vi "Calibrate load cells.vi"() -> (3 "Slope and Intercept":dbl[][](array[numeric]))   [LabVIEW 2015]
uses:
  <vilib>/Utility/file.llb/Write Delimited Spreadsheet (DBL).vi
  <vilib>/Analysis/NI_AALPro.lvlib
  <vilib>/gmath/NI_Gmath.lvlib
panel:
  out "Left Hindlimb":dbl[](array[numeric])
  out "Right Hindlimb":dbl[](array[numeric])
  out "Forelimb":dbl[](array[numeric])
  in  "?":bool
  in  "Tab Control":T1(tab)
  in  "200g":bool
  out "200g":dbl
  in  "100g":bool
  out "100g":dbl
  in  "50g":bool
  out "50g":dbl
  in  "OK Button":bool
  out "10g":dbl
  out "5g":dbl
  out "2g":dbl
  out "0g":dbl
  in  "20g":bool
  in  "15g":bool
  in  "10g":bool
  in  "2g":bool
  in  "0g":bool
  in  "5g":bool
  out "15g":dbl
  out "20g":dbl
  out "20g HR":dbl
  out "15g HR":dbl
  in  "5g HR":bool
  in  "0g HR":bool
  in  "2g HR":bool
  in  "10g HR":bool
  in  "15g HR":bool
  in  "20g HR":bool
  out "0g HR":dbl
  out "2g HR":dbl
  out "5g HR":dbl
  out "10g HR":dbl
  in  "OK Button 2":bool
  out "50g HR":dbl
  in  "50g HR":bool
  out "100g HR":dbl
  in  "100g HR":bool
  out "200g HR":dbl
  in  "200g HR":bool
  out "20g LH":dbl
  out "15g HL":dbl
  in  "5g HL":bool
  in  "0g HL":bool
  in  "2g HL":bool
  in  "10g HL":bool
  in  "15g HL":bool
  in  "20g HL":bool
  out "0g HL":dbl
  out "2g HL":dbl
  out "5g HL":dbl
  out "10g HL":dbl
  in  "OK Button 3":bool
  out "50g HL":dbl
  in  "50g HL":bool
  out "100g HL":dbl
  in  "100g HL":bool
  out "200g HL":dbl
  in  "200g HL":bool
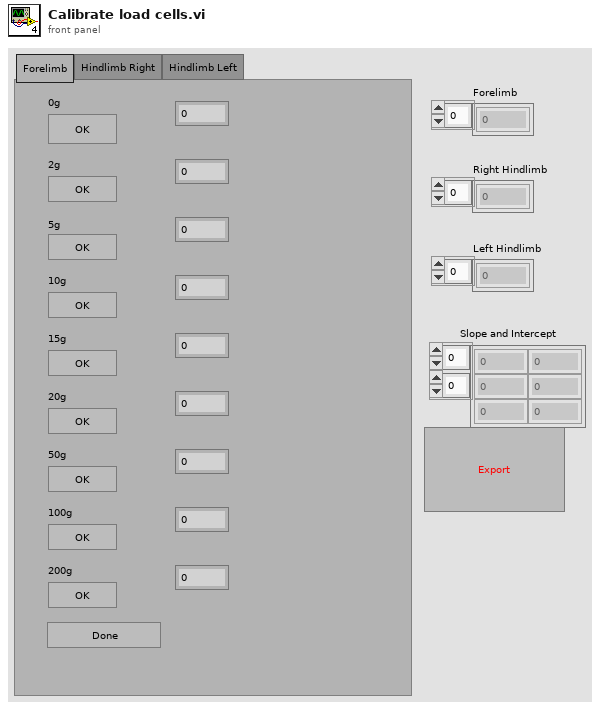
[diagram p1: front panel]
types:
  T1 = enum32{"Forelimb", "Hindlimb Right", "Hindlimb Left"}
  T2 = enum16{"arithmetic", "geometric", "harmonic", "trimmed", "median"}
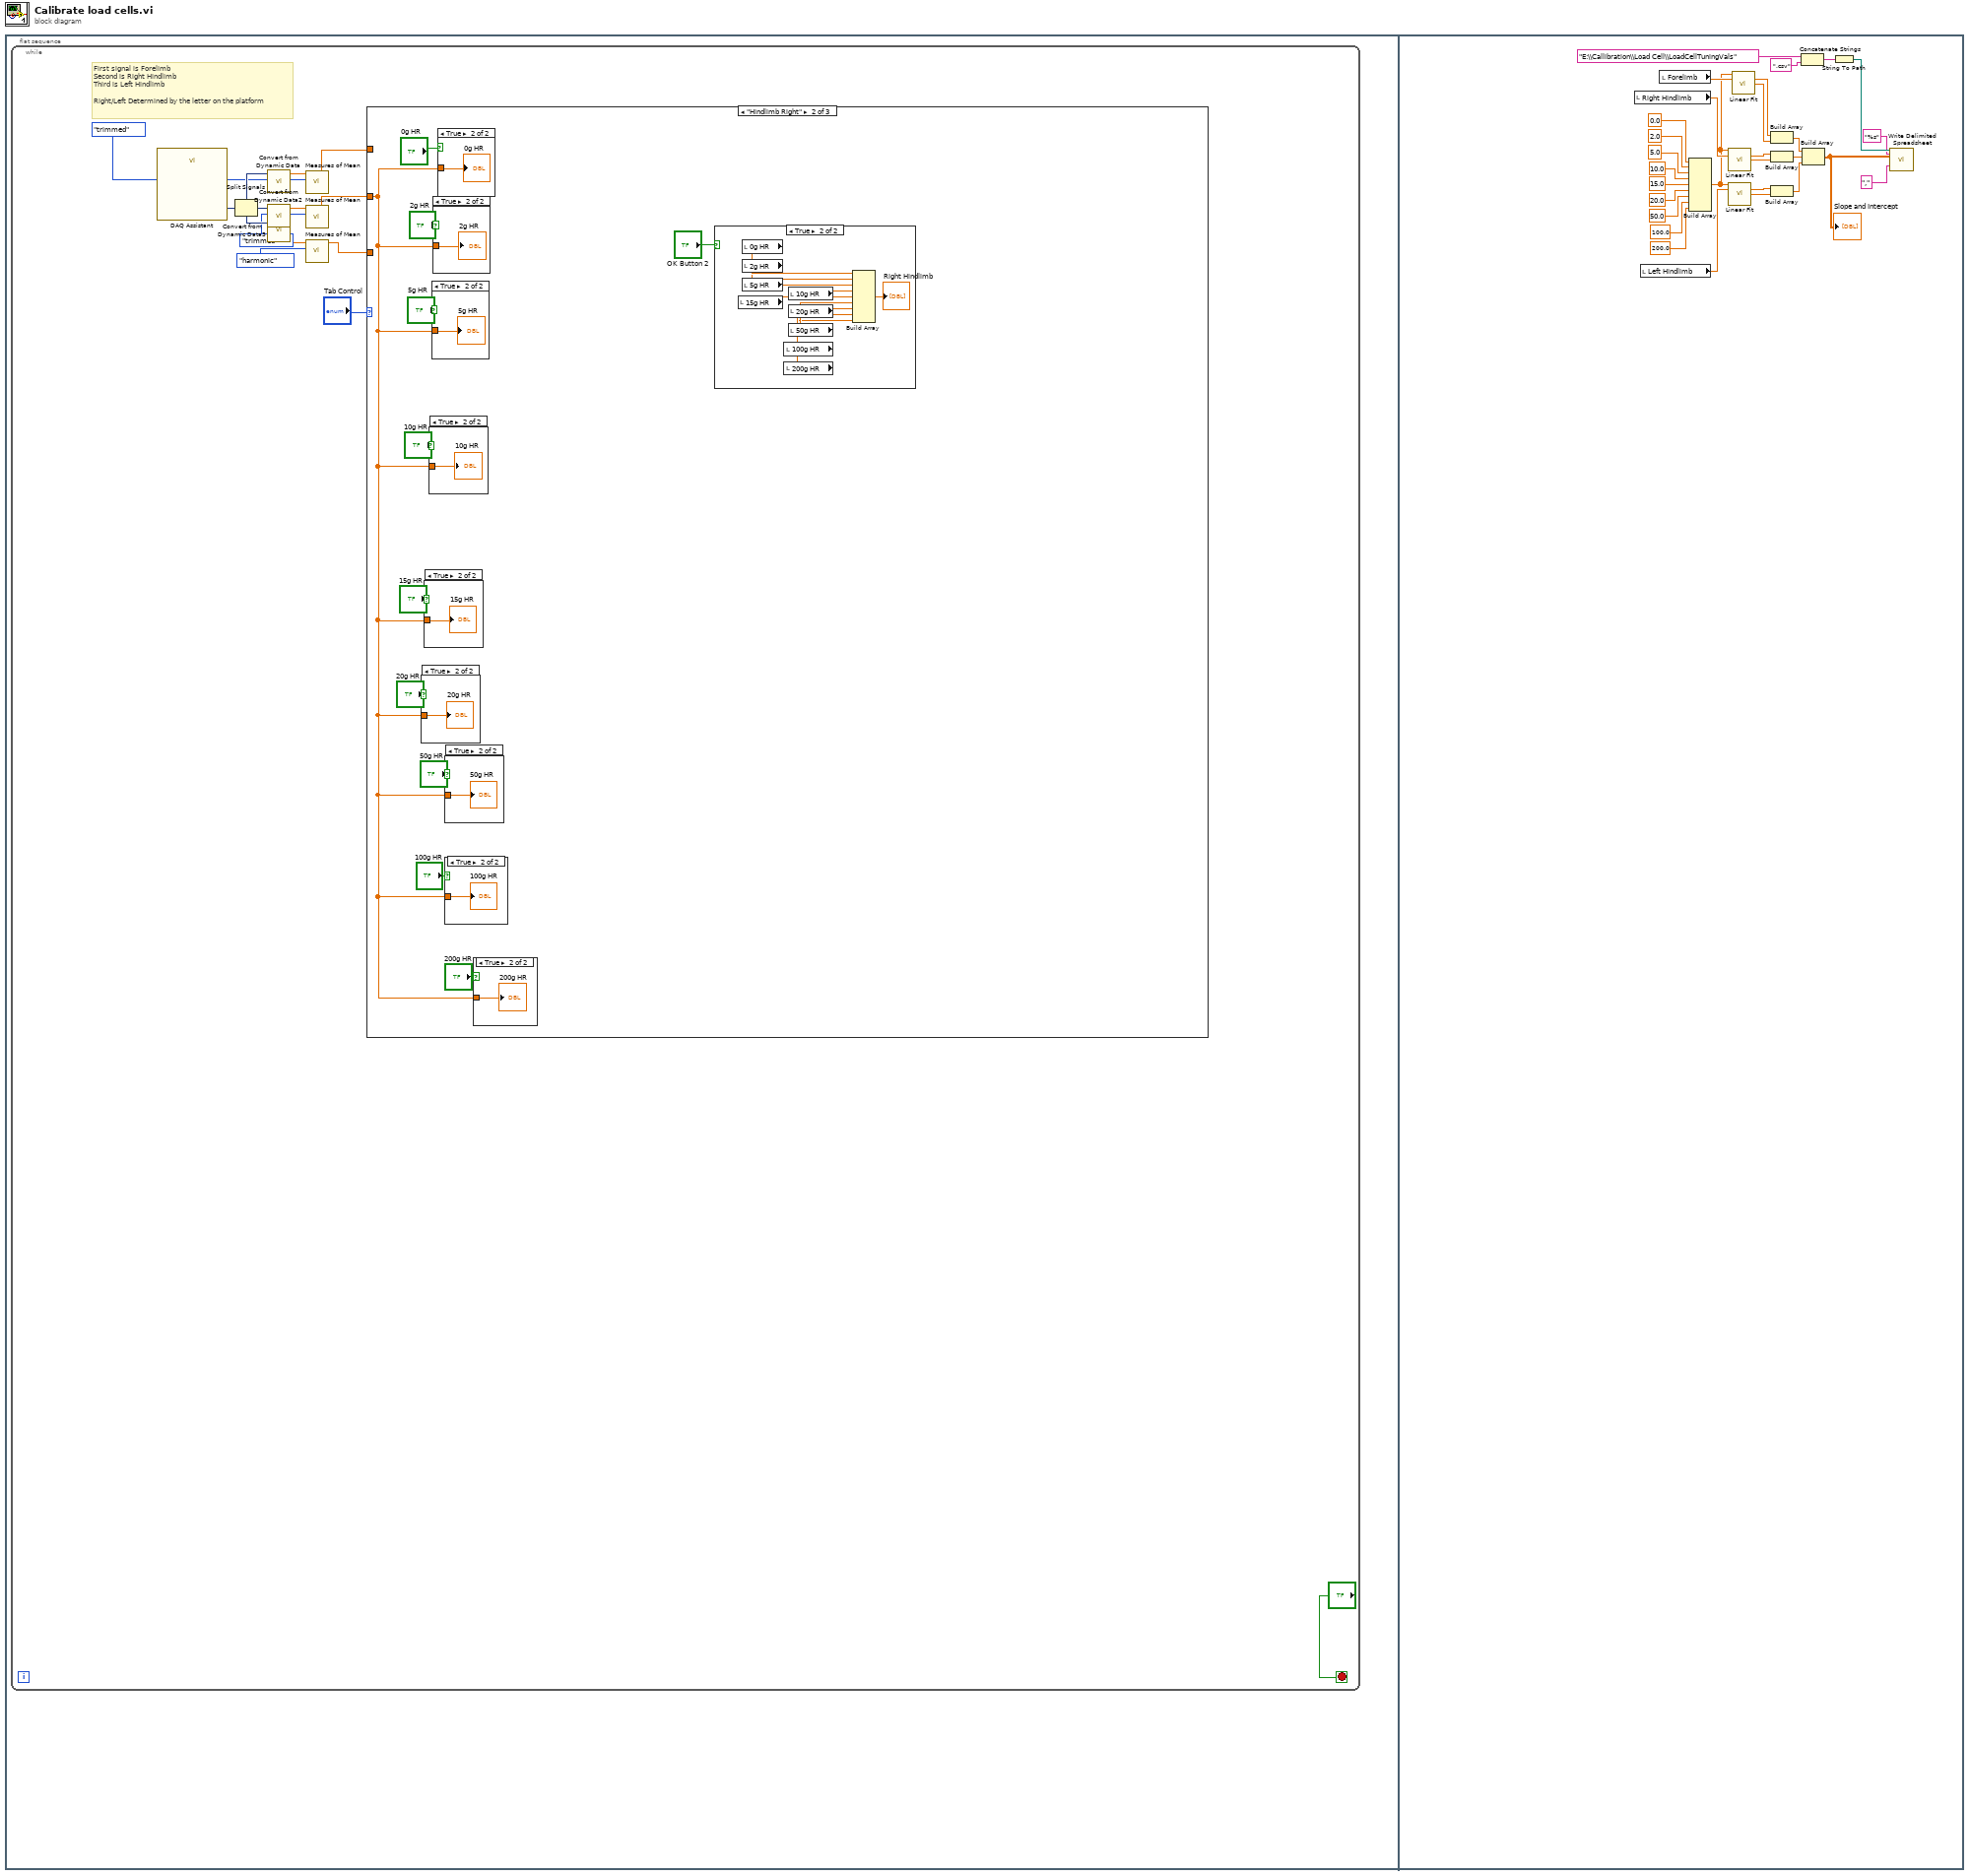
[diagram p0: block diagram]
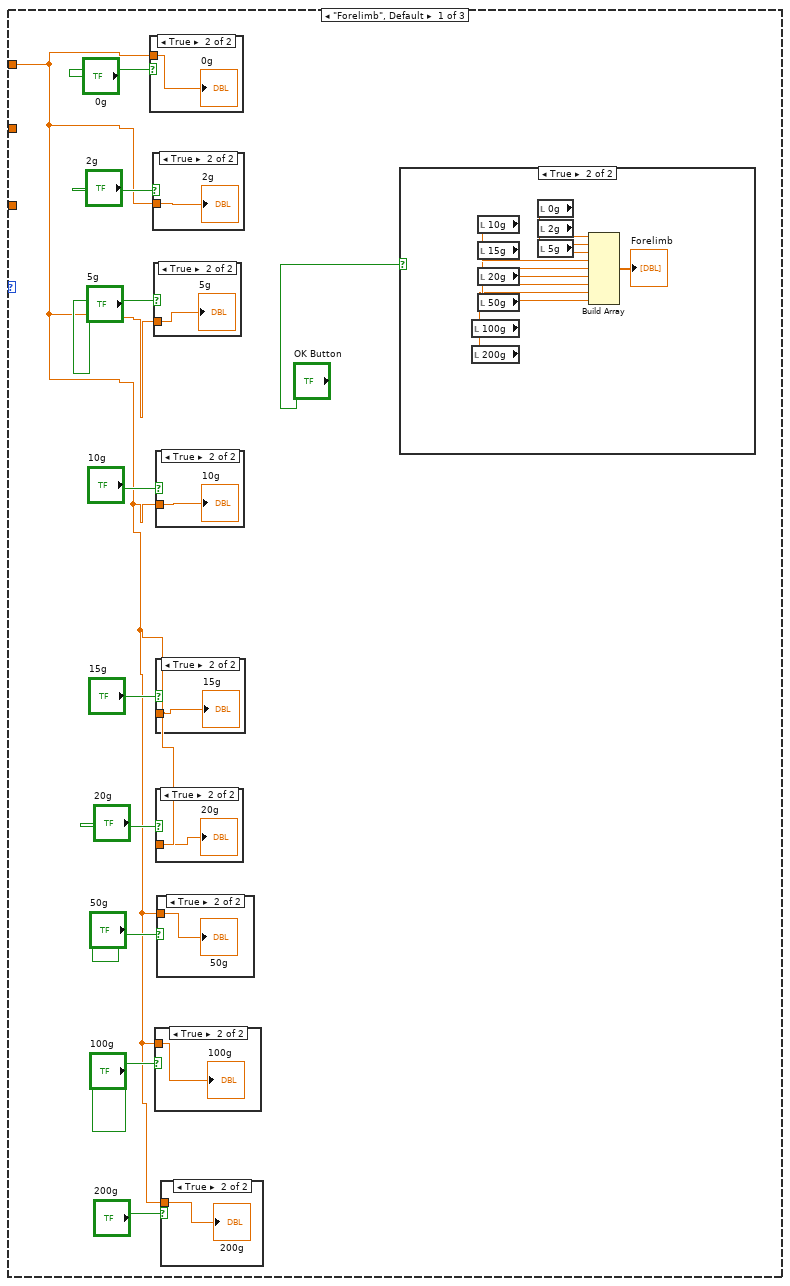
[diagram p2: hidden frame]
diagram:
  n1 = flat-sequence {
    frame #0 {
      n2 = while {
        stop <- "?" stop-if-true
        # "First signal is Forelimb\nSecond is Right Hindlimb\nThird is Left Hindlimb\n\nRight/Left Determined by the letter on the platform"
        n3 = call "DAQ Assistant"() -> ("data"=w7:dynamicdata)  [unwired: 17 in, 2 out]
        n4 = Split Signals(w7) -> (w15:dynamicdata, w13:dynamicdata, w11:dynamicdata)  [unwired: 3 in]
        n5 = call "Convert from Dynamic Data"("Dynamic Data Type"=w15) -> ("Array"=w14:dbl[])  [unwired: 3 in]
        n6 = call "Convert from Dynamic Data2"("Dynamic Data Type"=w13) -> ("Array"=w12:dbl[])  [unwired: 3 in]
        n7 = call "Convert from Dynamic Data3"("Dynamic Data Type"=w11) -> ("Array"=w6:dbl[])  [unwired: 3 in]
        n8 = call <vilib>:"Measures of Mean.vi"("type"=T2."trimmed", "x array"=w14) -> ("mean value"=w9:dbl)  [unwired: 8 in, 1 out]
        n9 = call <vilib>:"Measures of Mean.vi"("type"=T2."trimmed", "x array"=w12) -> ("mean value"=w2:dbl)  [unwired: 8 in, 1 out]
        n10 = call <vilib>:"Measures of Mean.vi"("type"=T2."harmonic", "x array"=w6) -> ("mean value"=w1:dbl)  [unwired: 8 in, 1 out]
        n11 = case shown="\"Hindlimb Right\"" "Tab Control" {
          tunnel: w9 -> [w16 _ _]
          tunnel: w1 -> [_ _ w76]
          tunnel: w2 -> [_ w46 _]
          frame "Forelimb", Default {
            n12 = case shown="True" "0g" {
              tunnel: w16 -> [_ w45]
              frame False {
              }
              frame True {
                "0g" <- w45
              }
            }
            n13 = case shown="True" "2g" {
              tunnel: w16 -> [_ w44]
              frame False {
              }
              frame True {
                "2g" <- w44
              }
            }
            n14 = case shown="True" "5g" {
              tunnel: w16 -> [_ w43]
              frame False {
              }
              frame True {
                "5g" <- w43
              }
            }
            n15 = case shown="True" "100g" {
              tunnel: w16 -> [_ w28]
              frame False {
              }
              frame True {
                "100g" <- w28
              }
            }
            n16 = case shown="True" "10g" {
              tunnel: w16 -> [_ w42]
              frame False {
              }
              frame True {
                "10g" <- w42
              }
            }
            n17 = case shown="True" "15g" {
              tunnel: w16 -> [_ w41]
              frame False {
              }
              frame True {
                "15g" <- w41
              }
            }
            n18 = case shown="True" "20g" {
              tunnel: w16 -> [_ w40]
              frame False {
              }
              frame True {
                "20g" <- w40
              }
            }
            n19 = case shown="True" "50g" {
              tunnel: w16 -> [_ w29]
              frame False {
              }
              frame True {
                "50g" <- w29
              }
            }
            n20 = case shown="True" "200g" {
              tunnel: w16 -> [_ w27]
              frame False {
              }
              frame True {
                "200g" <- w27
              }
            }
            n21 = case shown="True" "OK Button" {
              frame False {
              }
              frame True {
                n22 = local read "100g"() -> (w31:dbl)
                n23 = local read "200g"() -> (w30:dbl)
                n24 = local read "10g"() -> (w36:dbl)
                n25 = local read "15g"() -> (w35:dbl)
                n26 = local read "20g"() -> (w34:dbl)
                n27 = local read "50g"() -> (w32:dbl)
                n28 = local read "0g"() -> (w39:dbl)
                n29 = local read "2g"() -> (w38:dbl)
                n30 = local read "5g"() -> (w37:dbl)
                n31 = Build Array(w39, w38, w37, w36, w35, w34, w32, w31, w30) -> (→"Forelimb":dbl[])
              }
            }
          }
          frame "Hindlimb Right" {
            n32 = case shown="True" "20g HR" {
              tunnel: w46 -> [_ w70]
              frame False {
              }
              frame True {
                "20g HR" <- w70
              }
            }
            n33 = case shown="True" "15g HR" {
              tunnel: w46 -> [_ w71]
              frame False {
              }
              frame True {
                "15g HR" <- w71
              }
            }
            n34 = case shown="True" "10g HR" {
              tunnel: w46 -> [_ w72]
              frame False {
              }
              frame True {
                "10g HR" <- w72
              }
            }
            n35 = case shown="True" "5g HR" {
              tunnel: w46 -> [_ w73]
              frame False {
              }
              frame True {
                "5g HR" <- w73
              }
            }
            n36 = case shown="True" "2g HR" {
              tunnel: w46 -> [_ w74]
              frame False {
              }
              frame True {
                "2g HR" <- w74
              }
            }
            n37 = case shown="True" "0g HR" {
              tunnel: w46 -> [_ w75]
              frame False {
              }
              frame True {
                "0g HR" <- w75
              }
            }
            n38 = case shown="True" "50g HR" {
              tunnel: w46 -> [_ w59]
              frame False {
              }
              frame True {
                "50g HR" <- w59
              }
            }
            n39 = case shown="True" "100g HR" {
              tunnel: w46 -> [_ w58]
              frame False {
              }
              frame True {
                "100g HR" <- w58
              }
            }
            n40 = case shown="True" "200g HR" {
              tunnel: w46 -> [_ w57]
              frame False {
              }
              frame True {
                "200g HR" <- w57
              }
            }
            n41 = case shown="True" "OK Button 2" {
              frame False {
              }
              frame True {
                n42 = local read "15g HR"() -> (w65:dbl)
                n43 = local read "0g HR"() -> (w69:dbl)
                n44 = local read "2g HR"() -> (w68:dbl)
                n45 = local read "5g HR"() -> (w67:dbl)
                n46 = local read "100g HR"() -> (w61:dbl)
                n47 = local read "200g HR"() -> (w60:dbl)
                n48 = local read "10g HR"() -> (w66:dbl)
                n49 = local read "20g HR"() -> (w63:dbl)
                n50 = local read "50g HR"() -> (w62:dbl)
                n51 = Build Array(w69, w68, w67, w66, w65, w63, w62, w61, w60) -> (→"Right Hindlimb":dbl[])
              }
            }
          }
          frame "Hindlimb Left" {
            n52 = case shown="True" "0g HL" {
              tunnel: w76 -> [_ w105]
              frame False {
              }
              frame True {
                "0g HL" <- w105
              }
            }
            n53 = case shown="True" "2g HL" {
              tunnel: w76 -> [_ w104]
              frame False {
              }
              frame True {
                "2g HL" <- w104
              }
            }
            n54 = case shown="True" "5g HL" {
              tunnel: w76 -> [_ w103]
              frame False {
              }
              frame True {
                "5g HL" <- w103
              }
            }
            n55 = case shown="True" "10g HL" {
              tunnel: w76 -> [_ w102]
              frame False {
              }
              frame True {
                "10g HL" <- w102
              }
            }
            n56 = case shown="True" "15g HL" {
              tunnel: w76 -> [_ w101]
              frame False {
              }
              frame True {
                "15g HL" <- w101
              }
            }
            n57 = case shown="True" "100g HL" {
              tunnel: w76 -> [_ w88]
              frame False {
              }
              frame True {
                "100g HL" <- w88
              }
            }
            n58 = case shown="True" "50g HL" {
              tunnel: w76 -> [_ w89]
              frame False {
              }
              frame True {
                "50g HL" <- w89
              }
            }
            n59 = case shown="True" "20g HL" {
              tunnel: w76 -> [_ w100]
              frame False {
              }
              frame True {
                "20g LH" <- w100
              }
            }
            n60 = case shown="True" "200g HL" {
              tunnel: w76 -> [_ w87]
              frame False {
              }
              frame True {
                "200g HL" <- w87
              }
            }
            n61 = case shown="True" "OK Button 3" {
              frame False {
              }
              frame True {
                n62 = local read "10g HL"() -> (w96:dbl)
                n63 = local read "15g HL"() -> (w95:dbl)
                n64 = local read "20g LH"() -> (w94:dbl)
                n65 = local read "50g HL"() -> (w93:dbl)
                n66 = local read "0g HL"() -> (w99:dbl)
                n67 = local read "2g HL"() -> (w98:dbl)
                n68 = local read "5g HL"() -> (w97:dbl)
                n69 = local read "100g HL"() -> (w92:dbl)
                n70 = local read "200g HL"() -> (w91:dbl)
                n71 = Build Array(w99, w98, w97, w96, w95, w94, w93, w92, w91) -> (→"Left Hindlimb":dbl[])
              }
            }
          }
        }
      }
    }
    frame #1 {
      n72 = local read "Right Hindlimb"() -> (w111:dbl[])
      n73 = local read "Left Hindlimb"() -> (w109:dbl[])
      n74 = local read "Forelimb"() -> (w112:dbl[])
      n75 = Build Array(0.0 ("element"), 2.0 ("element"), 5.0 ("element"), 10.0 ("element"), 15.0 ("element"), 20.0 ("element"), 50.0 ("element"), 100.0 ("element"), 200.0 ("element")) -> (w110:dbl[])
      n76 = call <vilib>:"Linear Fit.vi"("Y"=w110, "X"=w111) -> ("slope"=w126:dbl, "intercept"=w125:dbl)  [unwired: 9 in, 3 out]
      n77 = call <vilib>:"Linear Fit.vi"("Y"=w110, "X"=w109) -> ("slope"=w124:dbl, "intercept"=w123:dbl)  [unwired: 9 in, 3 out]
      n78 = call <vilib>:"Linear Fit.vi"("Y"=w110, "X"=w112) -> ("slope"=w128:dbl, "intercept"=w127:dbl)  [unwired: 9 in, 3 out]
      n79 = Build Array(w128, w127) -> (w116:dbl[])
      n80 = Build Array(w126, w125) -> (w115:dbl[])
      n81 = Build Array(w124, w123) -> (w114:dbl[])
      n82 = Concatenate Strings("E:\\Callibration\\Load Cell\\LoadCellTuningVals" ("string"), ".csv" ("string")) -> (w121:string)
      n83 = Build Array(w116, w115, w114) -> (w113:dbl[][])
      "Slope and Intercept" <- w113
      n84 = String To Path(string=w121) -> (path=w119:path)
      n85 = call-poly <vilib>:"Write Delimited Spreadsheet.vi"("file path (dialog if empty)"=w119, "format (%.3f)"="%s" ("format (%s)"), "2D data"=w113, "delimiter (\\t)"="," ("delimiter (\\t)")) -> ()  [unwired: 10 in, 2 out]
    }
  }
